vi "Read Function Source.vi"(8 "error in (no error)":errorcluster, 10 "Function Channel (1: Function 1)":i32(ring)=1 items=["Function 1"=1, "Function 2"=2, "Function 3"=3, "Function 4"=4, "Function 5"=5, "Function 6"=6, "Function 7"=7, "Function 8"=8, "Function 9"=9, "Function 10"=10, "Function 11"=11, "Function 12"=12, "Function 13"=13, "Function 14"=14, "Function 15"=15, "Function 16"=16], 11 "VISA resource name":refnum<visa-resource-name>) -> (0 "error out":errorcluster, 1 "Function Source 2":string="0", 2 "Function Source 1":string="0", 3 "VISA resource name out":refnum<visa-resource-name>)   [LabVIEW 2020, in "Agilent 90000 Series.lvlib"]
doc: "Queries the currently defined source(s) for the function."
uses:
  Agilent 90000 Series.lvlib
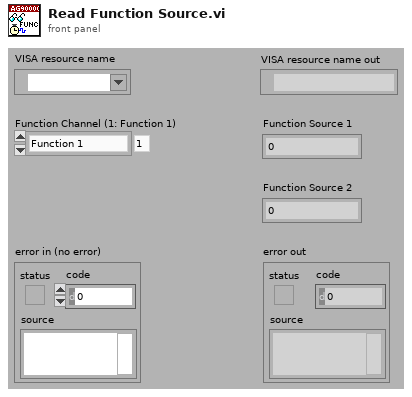
[diagram p1: front panel]
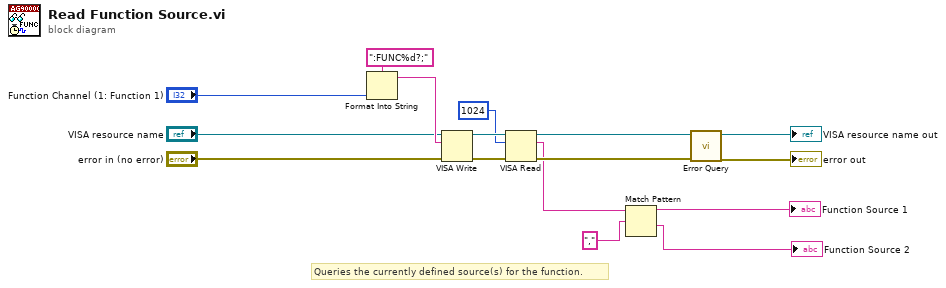
[diagram p0: block diagram]
diagram:
  # "Queries the currently defined source(s) for the function."
  n1 = Format Into String(format string=":FUNC%d?;", "Function Channel (1: Function 1)") -> (resulting string=w14:string)  [unwired: 2 in, 1 out]
  n2 = VISA Write(VISA resource name="VISA resource name", write buffer=w14, error in (no error)="error in (no error)") -> (VISA resource name out=w9:refnum<visa-resource-name>, error out=w8:errorcluster)  [unwired: 1 out]
  n3 = VISA Read(VISA resource name=w9, byte count=u32 1024, error in (no error)=w8) -> (VISA resource name out=w4:refnum<visa-resource-name>, read buffer=w1:string, error out=w3:errorcluster)  [unwired: 1 out]
  n4 = Match Pattern(string=w1, regular expression=",") -> (before substring=→"Function Source 1":string, after substring=→"Function Source 2":string)  [unwired: 1 in, 2 out]
  n5 = call "Error Query.vi"("error in (no error)"=w3, "VISA resource name"=w4) -> ("error out"=→"error out":errorcluster, "VISA resource name out"=→"VISA resource name out":refnum<visa-resource-name>)  [unwired: 6 in, 2 out]
